vi "Load Configuration.vi"(8 "error in":errorcluster) -> (0 "error out":errorcluster, 3 "Config DVR":refnum<data-value>)   [LabVIEW 2019]
uses:
  Controls/INI DataType.ctl
  Controls/KeyValue.ctl
  <vilib>/Utility/config.llb/Read Key (String).vi
  <vilib>/Utility/config.llb/NI_LVConfig.lvlib
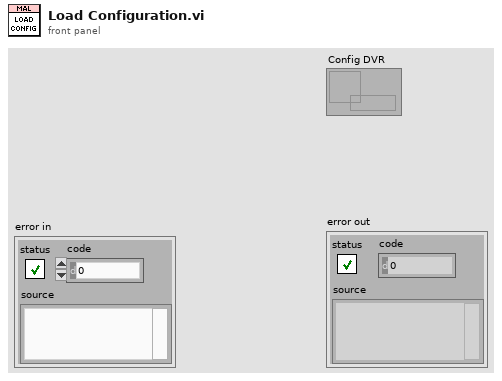
[diagram p1: front panel]
types:
  T1 = typedef "NI_LVConfig.lvlib/Config Data RefNum.ctl" = refnum<k1>
  T2 = typedef "INI DataType.ctl" = cluster{"Section":string, "Data":variant}
  T3 = typedef "KeyValue.ctl" = cluster{"Key":string, "Value":string}
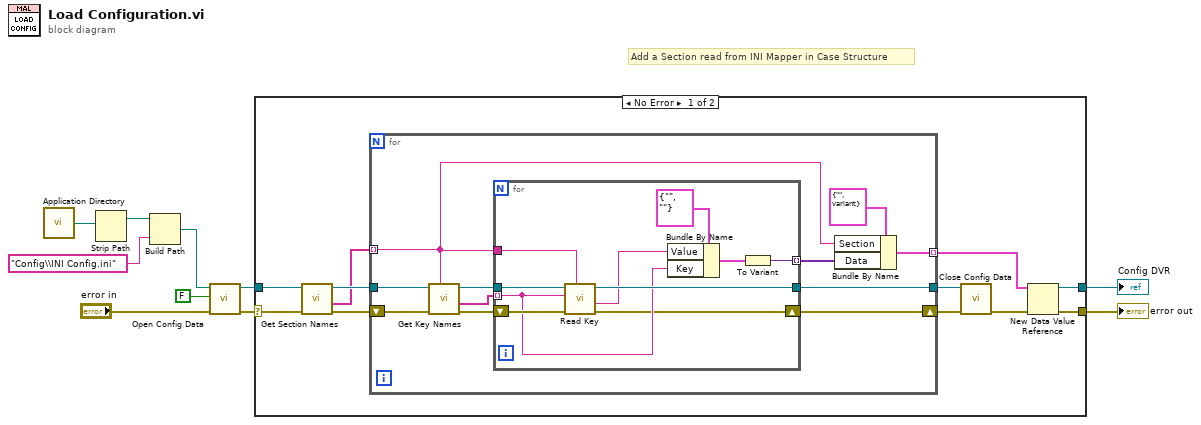
[diagram p0: block diagram]
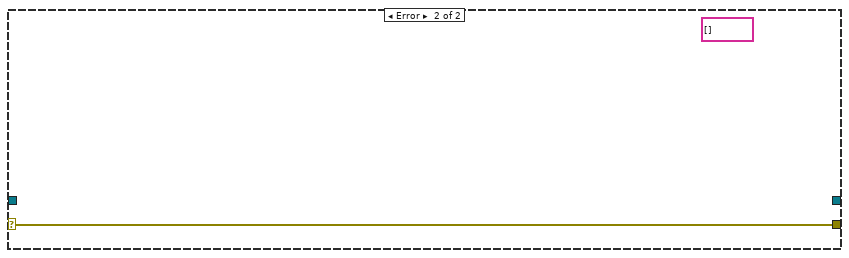
[diagram p2: hidden frame]
diagram:
  # "Add a Section read from INI Mapper in Case Structure"
  n1 = call <vilib>:"Application Directory.vi"() -> ("Application Directory"=w4:path)
  n2 = Strip Path(path=w4) -> (stripped path=w3:path)  [unwired: 1 out]
  n3 = Build Path(base path=w3, name or relative path="Config\\INI Config.ini") -> (appended path=w1:path)
  n4 = call <vilib>:"Open Config Data.vi"("error in (no error)"="error in", "create file if necessary (T)"=FALSE, "configuration file path"=w1) -> ("error out"=w8:errorcluster, "refnum"=w9:T1)  [unwired: 6 in, 1 out]
  n5 = case shown="No Error" w8 {
    selector: w8 -> [w21 w43]
    tunnel: [w13 w43] -> w6
    tunnel: w9 -> [w20 _]
    tunnel: [w12 _] -> w5
    frame No Error {
      n6 = call <vilib>:"Get Section Names.vi"("error in (no error)"=w21, "refnum"=w20) -> ("error out"=w19:errorcluster, "section names"=w11:string[], "refnum out"=w18:T1)  [unwired: 7 in]
      n7 = for {
        tunnel: w11 -> [w23] mode=indexing
        tunnel: w18 -> [w31]
        tunnel: [w30] -> w17
        shift-right: [w24] -> w16
        shift-left: w19 -> [w32]
        tunnel: [w26] -> w15 mode=indexing
        n8 = call <vilib>:"Get Key Names.vi"("section"=w23, "error in (no error)"=w32, "refnum"=w31) -> ("error out"=w29:errorcluster, "key names"=w28:string[], "refnum out"=w27:T1)  [unwired: 5 in, 1 out]
        n9 = for {
          tunnel: w28 -> [w35] mode=indexing
          tunnel: w23 -> [w39]
          tunnel: w27 -> [w41]
          tunnel: [w40] -> w30
          tunnel: [w36] -> w25 mode=indexing
          shift-right: [w34] -> w24
          shift-left: w29 -> [w42]
          n10 = call-poly <vilib>:"Read Key.vi"("section"=w39, "error in (no error)"=w42, "key"=w35, "refnum"=w41) -> ("error out"=w34:errorcluster, "value"=w37:string, "refnum out"=w40:T1)  [unwired: 4 in, 1 out]
          n11 = Bundle By Name(cluster=T3 {"Key"="", "Value"=""} ("INI Data"), "Value"=w37, "Key"=w35) -> (w38:T3)
          n12 = To Variant(anything=w38) -> (Variant=w36:variant)
        }
        n13 = Bundle By Name(cluster=T2 {"Section"="", "Data"=variant} ("INI Data Type"), "Section"=w23, "Data"=w25) -> (w26:T2)
      }
      n14 = call <vilib>:"Close Config Data.vi"("error in (no error)"=w16, "refnum"=w17) -> ("error out"=w14:errorcluster)  [unwired: 8 in, 1 out]
      n15 = New Data Value Reference(data value=w15, error in=w14) -> (data value reference=w12:refnum<data-value>, error out=w13:errorcluster)
    }
    frame Error {
      (unwired) string[] [] ("section names")
    }
  }
  "error out" <- w6
  "Config DVR" <- w5
